vi "OnDeviceSelected.vi"(8 "error in":errorcluster, 9 "Device Array":T2(array[cluster]), 10 "UI":T1, 11 "CmdLib In":refnum<k24>) -> (0 "error out":errorcluster)   [LabVIEW 2018]
uses:
  CmdLib.dll
  Global Variables.vi
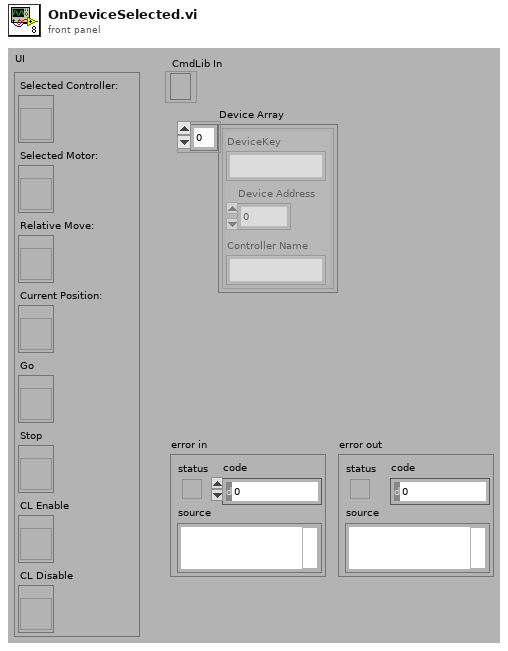
[diagram p1: front panel]
types:
  T1 = cluster{"Selected Controller:":refnum<vi>, "Selected Motor:":refnum<vi>, "Relative Move:":refnum<vi>, "Current Position:":refnum<vi>, "Go":refnum<vi>, "Stop":refnum<vi>, "CL Enable":refnum<vi>, "CL Disable":refnum<vi>}
  T2 = cluster{"DeviceKey":string, "Device Address":i32, "Controller Name":string}[]
  T3 = cluster{"DeviceKey":string, "Device Address":i32, "Controller Name":string}
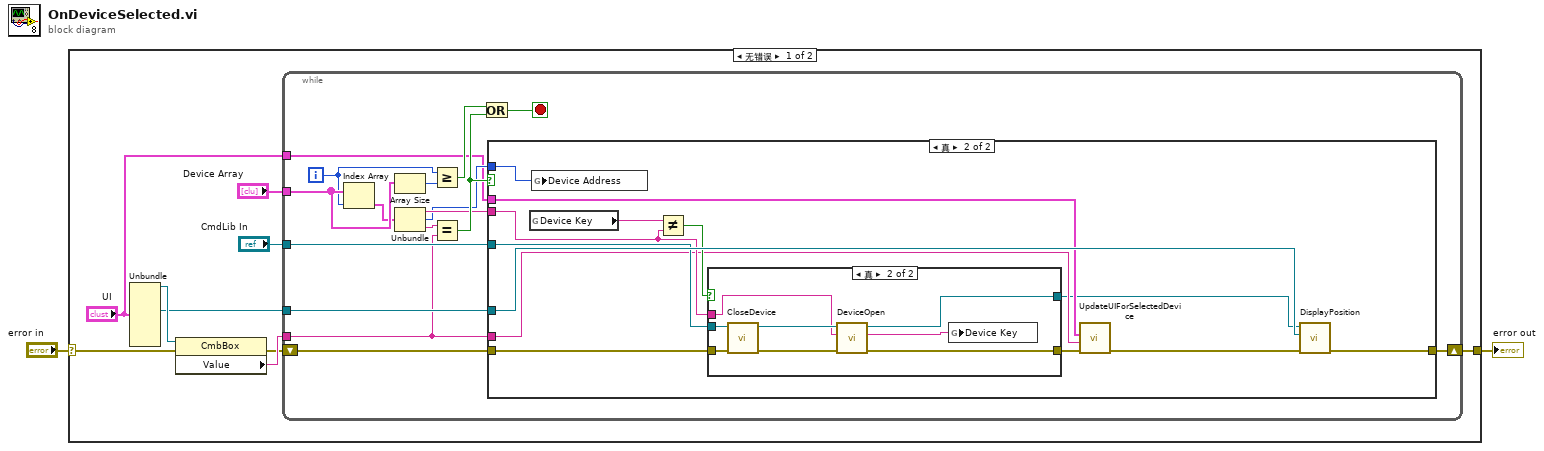
[diagram p0: block diagram]
diagram:
  n1 = case shown="无错误" "error in" {
    selector: "error in" -> [w8 w52]
    tunnel: [w10 w52] -> w2
    frame No Error {
      n2 = Unbundle("UI") -> ("Selected Controller:"=w5:refnum<vi>, "Current Position:"=w4:refnum<vi>)  [unwired: 6 out]
      n3 = property class="CmbBox"(reference=w5, error in=w8) -> (error out=w6:errorcluster, "Value"=w9:string)  [unwired: 1 out]
      n4 = while {
        tunnel: "Device Array" -> [w26]
        tunnel: w9 -> [w13]
        tunnel: w4 -> [w15]
        shift-right: [w17] -> w10
        shift-left: w6 -> [w16]
        tunnel: "CmdLib In" -> [w14]
        tunnel: "UI" -> [w12]
        i -> [w25]
        stop <- w20 stop-if-true
        n5 = Index Array(array=w26, index=w25) -> (element=w24:T3)
        n6 = Array Size(array=w26) -> (size(s)=w27:i32)
        n7 = Unbundle(w24) -> ("DeviceKey"=w19:string, "Device Address"=w18:i32, "Controller Name"=w23:string)
        n8 = Greater Or Equal?(x=w25, y=w27) -> (x >= y?=w22:bool)
        n9 = Equal?(x=w23, y=w13) -> (x = y?=w21:bool)
        n10 = Or(x=w22, y=w21) -> (x .or. y?=w20:bool)
        n11 = case shown="真" w21 {
          tunnel: w19 -> [_ w37]
          tunnel: w18 -> [_ w34]
          tunnel: [w28 w41] -> w17
          tunnel: w16 -> [w28 w39]
          tunnel: w15 -> [_ w40]
          tunnel: w14 -> [_ w35]
          tunnel: w13 -> [_ w31]
          tunnel: w12 -> [_ w30]
          frame False {
          }
          frame True {
            n12 = global read "Global Variables.vi" "Device Key"() -> (w38:string)
            n13 = global write "Global Variables.vi" "Device Address"(w34) -> ()
            n14 = Not Equal?(x=w38, y=w37) -> (x != y?=w36:bool)
            n15 = case shown="真" w36 {
              tunnel: [w43 w45] -> w33
              tunnel: w35 -> [w42 w51]
              tunnel: w39 -> [w43 w49]
              tunnel: w37 -> [_ w47]
              tunnel: [w42 w44] -> w29
              frame False {
              }
              frame True {
                n16 = call "CloseDevice.vi"("error in"=w49, "CmdLib In"=w51) -> ("error out"=w50:errorcluster, "CmdLib Out"=w48:refnum<k24>)  [unwired: 8 in]
                n17 = call "DeviceOpen.vi"("error in (no error)"=w50, "DeviceKey In"=w47, "CmdLib In"=w48) -> ("error out"=w45:errorcluster, "DeviceKey Out"=w46:string, "CmdLib Out"=w44:refnum<k24>)  [unwired: 2 in]
                n18 = global write "Global Variables.vi" "Device Key"(w46) -> ()
              }
            }
            n19 = call "UpdateUIForSelectedDevice.vi"("error in"=w33, "Controller Name"=w31, "UI"=w30) -> ("error out"=w32:errorcluster)  [unwired: 8 in]
            n20 = call "DisplayPosition.vi"("error in"=w32, "Current Position:"=w40, "CmdLib In"=w29) -> ("error out"=w41:errorcluster)  [unwired: 7 in, 1 out]
          }
        }
      }
    }
    frame Error {
    }
  }
  "error out" <- w2
